vi "aCKNOWLEDGE.vi"(8 "error in (no error)":errorcluster, 11 "Signal Acquisition in":refnum<class "Signal Acquisition.lvclass">) -> (0 "error out":errorcluster, 3 "Signal Acquisition out":refnum<class "Signal Acquisition.lvclass">)   [LabVIEW 2022 SP3, in "Signal Acquisition.lvlib" / "Signal Acquisition.lvclass"]
uses:
  Signal Acquisition.lvclass
  Signal Acquisition.lvclass/Signal Acquisition.ctl
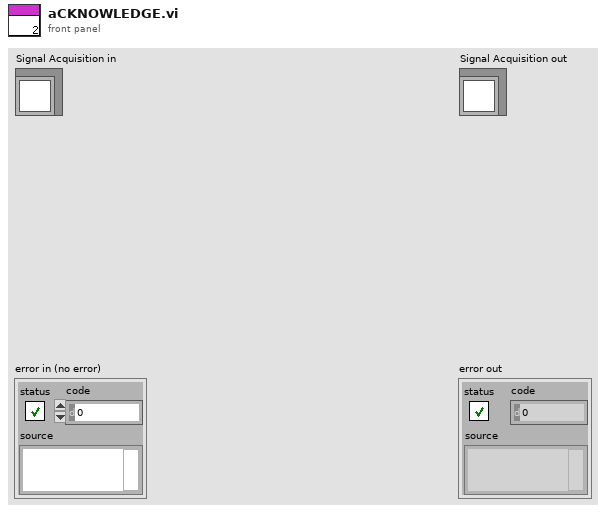
[diagram p1: front panel]
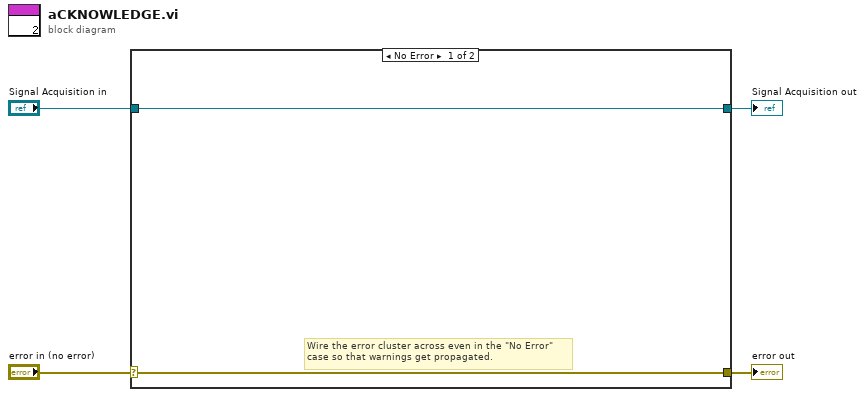
[diagram p0: block diagram]
diagram:
  n1 = case shown="No Error" "error in (no error)" {
    selector: "error in (no error)" -> [w5 w8]
    tunnel: [w5 w8] -> w3
    tunnel: [w6 w7] -> w1
    tunnel: "Signal Acquisition in" -> [w6 w7]
    frame No Error {
      # "Wire the error cluster across even in the \"No Error\"\ncase so that warnings get propagated."
    }
    frame Error {
    }
  }
  "error out" <- w3
  "Signal Acquisition out" <- w1
